vi "FPGA Counts.vi"(0 "saveData":bool, 2 "runs":i32, 5 "fpgaCommand":u8, 7 "fileName":string, 11 "error in (no error)":errorcluster) -> (4 "function return":i32, 8 "fileName out":string, 12 "Data":u64[](array[numeric]), 13 "Stats":i64[](array[numeric]), 14 "length out":i32, 15 "error out":errorcluster)   [LabVIEW 2012, in "Stats32.lvlib"]
doc: "LIBRARY_API int FPGA_Counts(bool saveData, unsigned char fpgaCommand, char* fileName, int* stats, unsigned int* data, int* length, int runs);"
uses:
  Stats32.lvlib
  Stats/Release/Win32/Stats32.dll
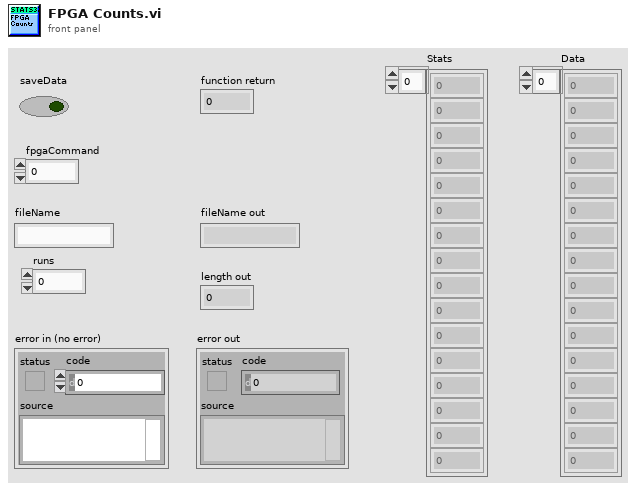
[diagram p1: front panel]
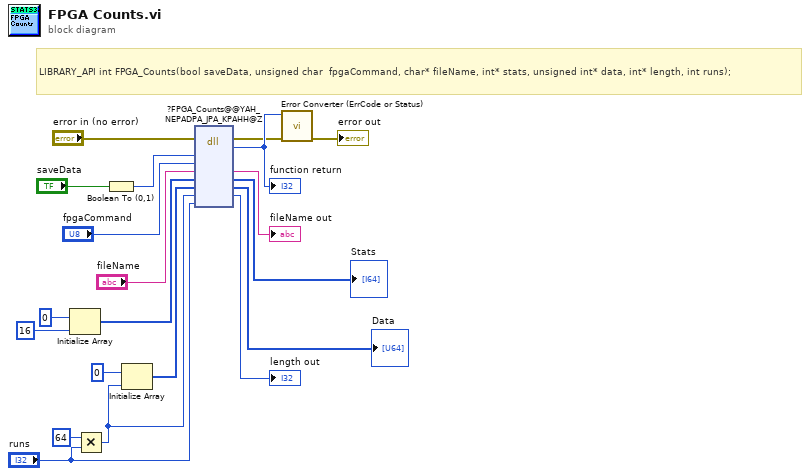
[diagram p0: block diagram]
diagram:
  # "LIBRARY_API int FPGA_Counts(bool saveData, unsigned char  fpgaCommand, char* fileName, int* stats, unsigned int* data, int* length, int runs);"
  n1 = Initialize Array(0, 16) -> (w3:i32[])
  n2 = Multiply(x=64, y="runs") -> (x*y=w8:i32)
  n3 = Boolean To (0,1)(Boolean="saveData") -> (0, 1=w18:i16)
  n4 = Initialize Array(0, w8) -> (w6:i32[])
  n5 = dll-call lib="C:/Programming/Stats/Stats/Release/Win32/Stats32.*" fn="?FPGA_Counts@@YAH_NEPADPA_JPA_KPAHH@Z"(error in="error in (no error)", "saveData"=w18, "fpgaCommand"="fpgaCommand", "fileName"="fileName", "stats"=w3, "data"=w6, "length"=w8, "runs"="runs") -> (error out=w12:errorcluster, "return type"=w20:i32, "fileName"=→"fileName out":string, "stats"=→"Stats":i64[], "data"=→"Data":u64[], "length"=→"length out":i32)  [unwired: 5 in, 1 out]
  "function return" <- w20
  n6 = call "Error Converter (ErrCode or Status).vi"("error in (no error)"=w12, "error code"=w20) -> ("error out"=→"error out":errorcluster)  [unwired: 9 in]
